vi "Stop Core.vi"(10 "final error code":i32, 11 "Particle Counter in":refnum<class "Particle Counter.lvclass">) -> (3 "Particle Counter out":refnum<class "Particle Counter.lvclass">)   [LabVIEW 2023, in "Particle Counter.lvlib" / "Particle Counter.lvclass"]
doc: "(<B>Filename</B>: Actor Framework.lvlib:Actor.lvclass:Stop Core.vi)\n\nDefines what the actor does before it stops. Use the <B>final error code</B> input to determine whether the actor shut down in response to an error.\n\nBy default, this method passes the Stop message along to all auto-stop nested actors. A descendant class may override this method to define additional behavior, such as shutting down any processes the actor initiated in its override of the Actor Core method."
uses:
  Particle Counter.lvclass
  Particle Counter.lvclass/Particle Counter.ctl
  <vilib>/ActorFramework/Actor/Actor.lvclass
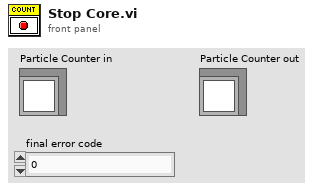
[diagram p1: front panel]
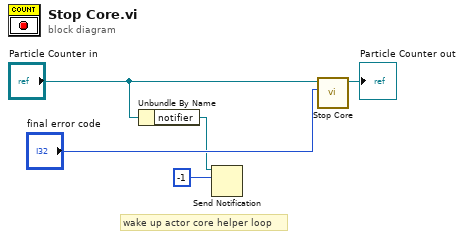
[diagram p0: block diagram]
diagram:
  # "wake up actor core helper loop"
  n1 = Unbundle By Name("Particle Counter in") -> ("notifier"=w2:refnum<notifier>)
  n2 = Send Notification(notification=-1, notifier=w2) -> ()  [unwired: 1 in, 2 out]
  n3 = call-parent "Stop Core.vi"("final error code"="final error code", "Actor in"="Particle Counter in") -> ("Actor out"=→"Particle Counter out":refnum<class "Particle Counter.lvclass">)  [unwired: 9 in]
